vi "Set Waveform Sweep Status.vi"(8 "error in (no error)":errorcluster, 10 "sweep status":T1, 11 "Waveforms in":waveform(dbl)[](array[waveform])) -> (0 "error out":errorcluster, 3 "Waveforms out":waveform(dbl)[](array[waveform]))   [LabVIEW 2019, in "Generator.lvclass"]
uses:
  Generator.lvclass
  typedefs/Generator.Sweep Status--enum.ctl
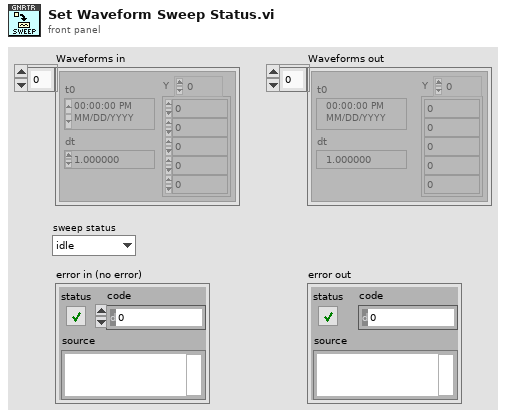
[diagram p1: front panel]
types:
  T1 = typedef "Generator.lvclass/Generator.Sweep Status--enum.ctl" = enum16{"idle", "initializing", "waiting", "sweeping", "stopping"}
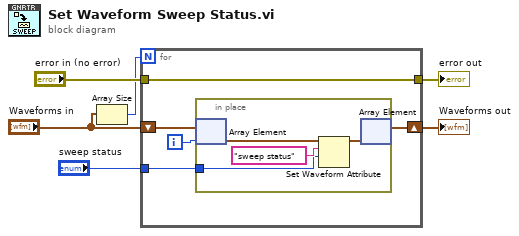
[diagram p0: block diagram]
diagram:
  n1 = Array Size(array="Waveforms in") -> (size(s)=w1:i32)
  n2 = for {
    N: w1 -> [_]
    shift-right: [w9] -> w3
    shift-left: "Waveforms in" -> [w10]
    tunnel: "error in (no error)" -> [w8]
    tunnel: [w8] -> w5
    tunnel: "sweep status" -> [w7]
    i -> [w11]
    n3 = in-place {
      in-place-border: w7 -> [w12]
      n4 = in-place-array #1(w10, w11) -> (w14:waveform(dbl))
      n5 = Set Waveform Attribute(5:w12, 6:"sweep status" ("name"), 7:w14) -> (3:w13:waveform(dbl))  [unwired: 1 in, 2 out]
      n6 = in-place-array #1(w13) -> (w9:waveform(dbl)[])  [unwired: 1 out]
    }
  }
  "error out" <- w5
  "Waveforms out" <- w3
